vi "PID Control Input Filter.vi"   [LabVIEW 2020, in "NI_PID_pid.lvlib"]
doc: "Applies a fifth-order lowpass finite impulse response (FIR) filter to the input value. Filter cut-off frequency is designed to be 1/10 of the sample frequency of the input value. Use this VI to filter measured values, such as the process variable, in control applications. Use the DBL instance of this VI to implement a single control loop. Use the DBL Array instance to implement parallel multi-loop control."
uses:
  NI_PID_pid.lvlib
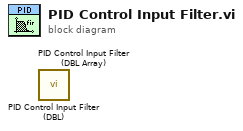
[diagram p0: block diagram]
diagram:
  n1 = call "PID Control Input Filter (DBL).vi"() -> ()  [unwired: 5 in, 1 out]
  n2 = call "PID Control Input Filter (DBL Array).vi"() -> ()  [unwired: 5 in, 1 out]
